vi "is_finished.vi"(8 "error in (no error)":errorcluster, 11 "ImagingModeDL100901FlexTrajectory in":refnum<class "ImagingModeDL100901FlexTrajectory.lvclass">) -> (0 "error out":errorcluster, 2 "finished?":bool[](array[boolean]), 3 "ImagingModeDL100901FlexTrajectory out":refnum<class "ImagingModeDL100901FlexTrajectory.lvclass">)   [LabVIEW 2010, in "ImagingModeDL100901FlexTrajectory.lvclass"]
uses:
  ImagingModeDL100901FlexTrajectory.lvclass
  ImagingModeDL100901FlexTrajectory.lvclass/ImagingModeDL100901FlexTrajectory.ctl
panel:
  # "element 0: is sweep finished?\n(further elements might be defined by overriding methods)"
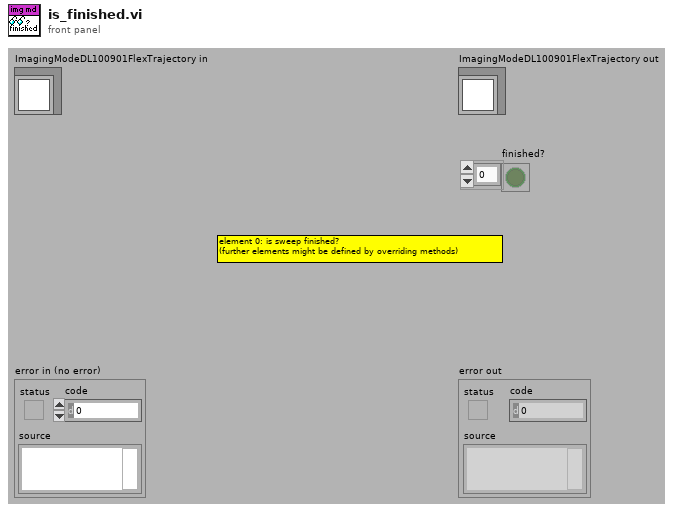
[diagram p1: front panel]
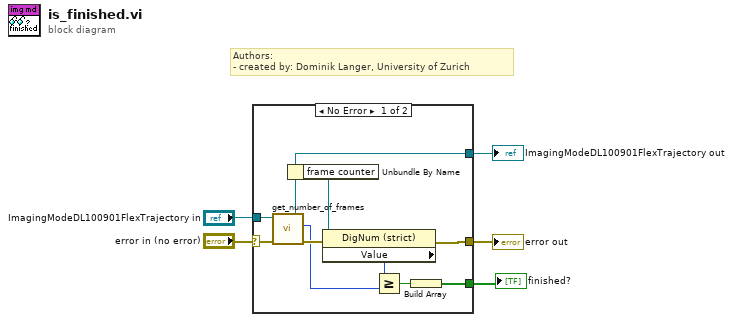
[diagram p0: block diagram]
diagram:
  # "Authors: \n- created by: Dominik Langer, University of Zurich"
  n1 = case shown="No Error" "error in (no error)" {
    selector: "error in (no error)" -> [w13 w16]
    tunnel: "ImagingModeDL100901FlexTrajectory in" -> [w15 w17]
    tunnel: [w10 w16] -> w3
    tunnel: [w14 w17] -> w2
    tunnel: [w6 _] -> w1
    frame No Error {
      n2 = call-dynamic "get_number_of_frames.vi"("error in (no error)"=w13, "ImagingModeDL100901FlexTrajectory in"=w15) -> ("error out"=w11:errorcluster, "number of frames"=w8:i32, "ImagingModeDL100901FlexTrajectory out"=w14:refnum<class "ImagingModeDL100901FlexTrajectory.lvclass">)  [unwired: 7 in]
      n3 = Unbundle By Name(w14) -> ("frame counter"=w12:refnum<vi>)
      n4 = property class="DigNum (strict)"(reference=w12, error in=w11) -> (error out=w10:errorcluster, "Value"=w9:i32)  [unwired: 1 out]
      n5 = Greater Or Equal?(x=w9, y=w8) -> (x >= y?=w7:bool)
      n6 = Build Array(w7) -> (w6:bool[])
    }
    frame Error {
    }
  }
  "error out" <- w3
  "ImagingModeDL100901FlexTrajectory out" <- w2
  "finished?" <- w1
